vi "Square.vi"(0 "Left":i32=210, 5 "Right":i32=205, 7 "Top":i32=200, 9 "Bottom":i32=200, 11 "error in (no error)":errorcluster) -> (15 "error out":errorcluster)   [LabVIEW 2017]
doc: "To draw a square box on the spherical object."
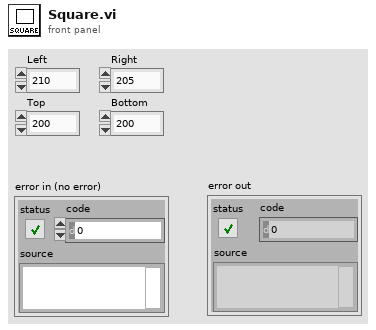
[diagram p1: front panel]
types:
  T1 = enum16{"Full", "Half", "Quarter", "Eighth", "Sixteenth"}
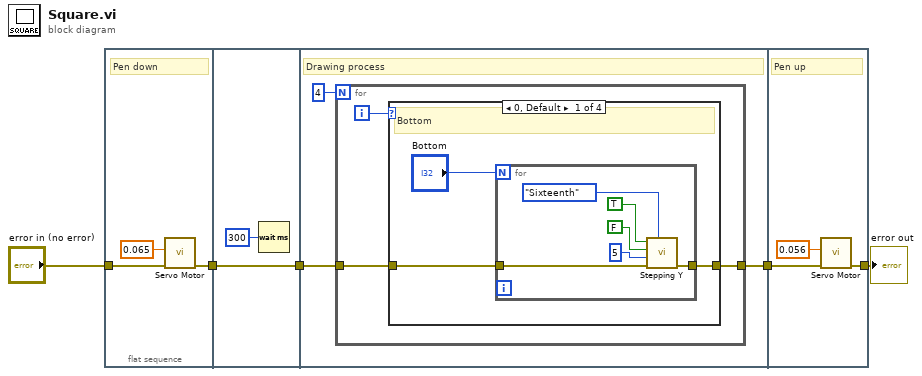
[diagram p0: block diagram]
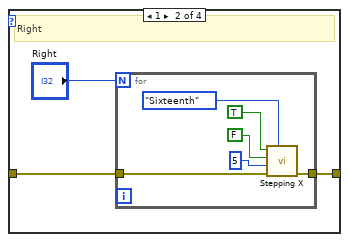
[diagram p2: hidden frame]
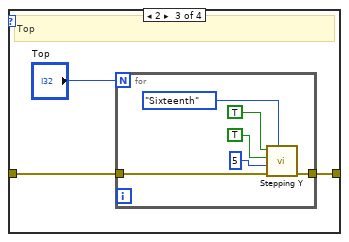
[diagram p3: hidden frame]
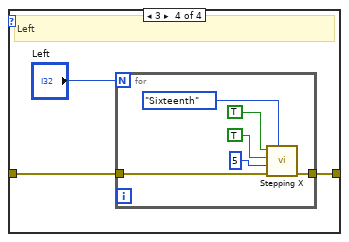
[diagram p4: hidden frame]
diagram:
  n1 = flat-sequence {
    tunnel: [w7] -> w2
    tunnel: "error in (no error)" -> [w6]
    tunnel: w2 -> [w10]
    tunnel: [w10] -> w1
    tunnel: [w12] -> w5
    tunnel: w1 -> [w11]
    tunnel: w5 -> [w54]
    tunnel: [w53] -> w3
    frame #0 {
      # "Pen down"
      n2 = call "Servo Motor.vi"("error in (no error)"=w6, "Duty Cycle"=0.065) -> ("error out"=w7:errorcluster)  [unwired: 9 in]
    }
    frame #1 {
      n3 = Wait (ms)(milliseconds to wait=u32 300) -> ()  [unwired: 1 out]
    }
    frame #2 {
      # "Drawing process"
      n4 = for {
        N: 4 -> [_]
        tunnel: [w15] -> w12
        tunnel: w11 -> [w14]
        i -> [w16]
        n5 = case shown="0, Default" w16 {
          tunnel: [w18 w26 w35 w44] -> w15
          tunnel: w14 -> [w17 w27 w36 w45]
          frame 0, Default {
            # "Bottom"
            n6 = for {
              N: "Bottom" -> [_]
              tunnel: [w21] -> w18
              tunnel: w17 -> [w20]
              n7 = call "Stepping Y.vi"("Microstep size"=T1."Sixteenth" ("Microstep size 2"), "error in (no error)"=w20, "Delay"=u32 5 ("Speed 2"), "Direction"=FALSE, "Enable"=TRUE) -> ("error out"=w21:errorcluster)  [unwired: 6 in]
            }
          }
          frame 1 {
            # "Right"
            n8 = for {
              N: "Right" -> [_]
              tunnel: [w30] -> w26
              tunnel: w27 -> [w29]
              n9 = call "Stepping X.vi"("Microstep size"=T1."Sixteenth", "error in (no error)"=w29, "Delay"=u32 5 ("Speed"), "Direction"=FALSE, "Enable"=TRUE) -> ("error out"=w30:errorcluster)  [unwired: 6 in]
            }
          }
          frame 2 {
            # "Top"
            n10 = for {
              N: "Top" -> [_]
              tunnel: [w39] -> w35
              tunnel: w36 -> [w38]
              n11 = call "Stepping Y.vi"("Microstep size"=T1."Sixteenth" ("Microstep size 2"), "error in (no error)"=w38, "Delay"=u32 5 ("Speed 2"), "Direction"=TRUE, "Enable"=TRUE) -> ("error out"=w39:errorcluster)  [unwired: 6 in]
            }
          }
          frame 3 {
            # "Left"
            n12 = for {
              N: "Left" -> [_]
              tunnel: [w48] -> w44
              tunnel: w45 -> [w47]
              n13 = call "Stepping X.vi"("Microstep size"=T1."Sixteenth", "error in (no error)"=w47, "Delay"=u32 5 ("Speed"), "Direction"=TRUE, "Enable"=TRUE) -> ("error out"=w48:errorcluster)  [unwired: 6 in]
            }
          }
        }
      }
    }
    frame #3 {
      # "Pen up"
      n14 = call "Servo Motor.vi"("error in (no error)"=w54, "Duty Cycle"=0.056) -> ("error out"=w53:errorcluster)  [unwired: 9 in]
    }
  }
  "error out" <- w3
